vi "UIRefs State.vi"(8 "error in (no error)":errorcluster, 11 "TCP 380 in":refnum<class "TCP 380.lvclass">) -> (0 "error out":errorcluster, 3 "TCP 380 out":refnum<class "TCP 380.lvclass">)   [LabVIEW 2021, in "TCP 380.lvlib" / "TCP 380.lvclass"]
uses:
  TCP 380.lvclass
  TCP 380.lvclass/TCP 380.ctl
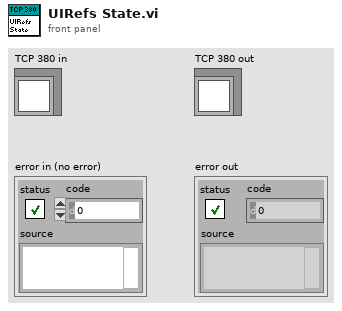
[diagram p1: front panel]
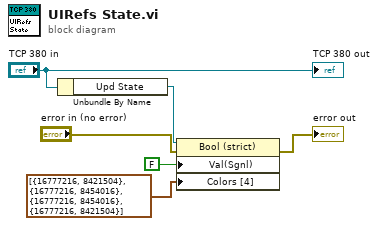
[diagram p0: block diagram]
diagram:
  n1 = Unbundle By Name("TCP 380 in") -> ("Upd State"=w5:refnum<vi>)
  n2 = property class="Bool (strict)"(reference=w5, error in="error in (no error)", "Val(Sgnl)"=FALSE ("Value (Signaling)"), "Colors [4]"=cluster{u32, u32}[] [{16777216, 8421504}, {16777216, 8454016}, {16777216, 8454016}, {16777216, 8421504}]) -> (error out=→"error out":errorcluster)  [unwired: 1 out]
  "TCP 380 out" <- "TCP 380 in"
